vi "boiler system open.vi"(8 "error in":errorcluster) -> (0 "error out":errorcluster, 2 "Notfilers":T2, 3 "Message Queues out":T1, 5 "Stop Event Registration Refnum":refnum<event-registration>, 7 "User Event - Stop":refnum<user-event>)   [LabVIEW 2015]
uses:
  Message Queue/All Message Queues.ctl
  Message Queue/Message Cluster.ctl
  Message Queue/Message Queue.lvlib
  User Event - Stop/User Event - Stop.lvlib
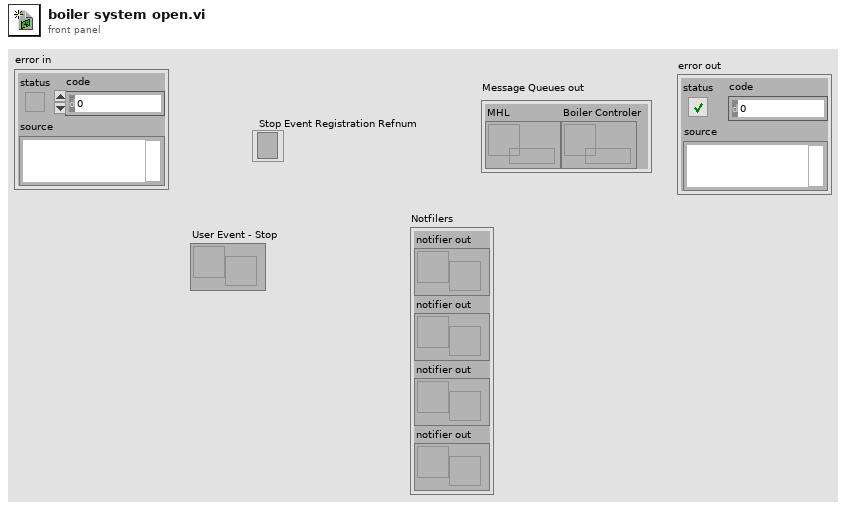
[diagram p1: front panel]
types:
  T1 = typedef "Message Queue.lvlib/All Message Queues.ctl" = cluster{"MHL":refnum<queue>, "Boiler Controler":refnum<queue>}
  T2 = cluster{"notifier out":refnum<notifier>, "notifier out":refnum<notifier>, "notifier out":refnum<notifier>, "notifier out":refnum<notifier>}
  T3 = typedef "Notifire.ctl" = cluster{"Handshake":refnum<notifier>, "Flame Level":refnum<notifier>, "Controller ":refnum<notifier>, "Boiler Exit":refnum<notifier>}
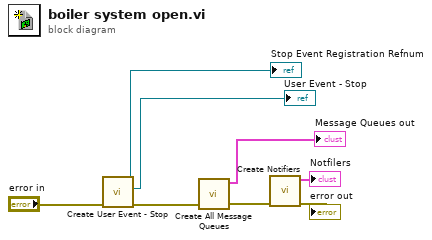
[diagram p0: block diagram]
diagram:
  n1 = call "Create User Event - Stop.vi"("error in (no error)"="error in") -> ("error out"=w8:errorcluster, "User bool - Stop"=→"User Event - Stop":refnum<user-event>, "Event Registration Refnum"=→"Stop Event Registration Refnum":refnum<event-registration>)  [unwired: 8 in]
  n2 = call "Create All Message Queues.vi"("error in (no error)"=w8) -> ("error out"=w6:errorcluster, "Message Queues out"=→"Message Queues out":T1)  [unwired: 9 in]
  n3 = call "Create Notifiers.vi"("error in"=w6) -> ("error out"=→"error out":errorcluster, "output cluster"=→"Notfilers":T3)  [unwired: 9 in]
